vi "DockVI.vi"(8 "ErrorIn":errorcluster, 10 "PanelVIRef":refnum<vi>, 11 "SubPanelIn":refnum<vi>) -> (0 "ErrorOut":errorcluster)   [LabVIEW 2021, in "MasterGUI.lvclass"]
uses:
  MasterGUI.lvclass
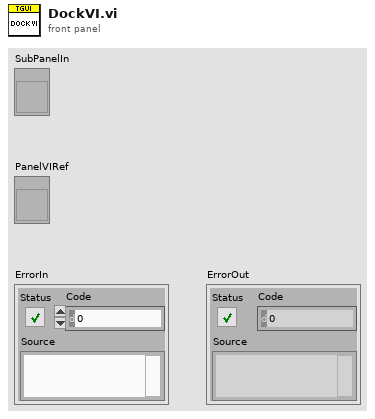
[diagram p1: front panel]
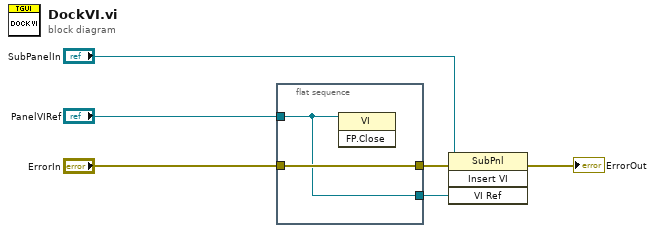
[diagram p0: block diagram]
diagram:
  n1 = flat-sequence {
    tunnel: "PanelVIRef" -> [w7]
    tunnel: "ErrorIn" -> [w8]
    tunnel: [w8] -> w6
    tunnel: [w7] -> w3
    frame #0 {
      n2 = invoke class="VI" method="FP.Close"(reference=w7) -> ()  [unwired: 2 in, 3 out]
    }
  }
  n3 = invoke class="SubPnl" method="Insert VI"(reference="SubPanelIn", error in=w6, "VI Ref"=w3) -> (error out=→"ErrorOut":errorcluster)  [unwired: 1 in, 3 out]
